vi "plot_displacement.vi"(6 "Position at Peak (decimicrons)":dbl, 7 "Target Pulse Duration (ms)":dbl, 9 "Array":dbl[](array[numeric]), 10 "Array 2":u32[](array[numeric]), 11 "XYGraph in":refnum<vi>) -> (1 "true pulse duration":dbl, 3 "Cluster":cluster{u32[], dbl[]})   [LabVIEW 2014]
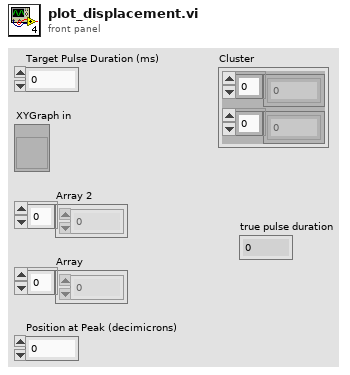
[diagram p1: front panel]
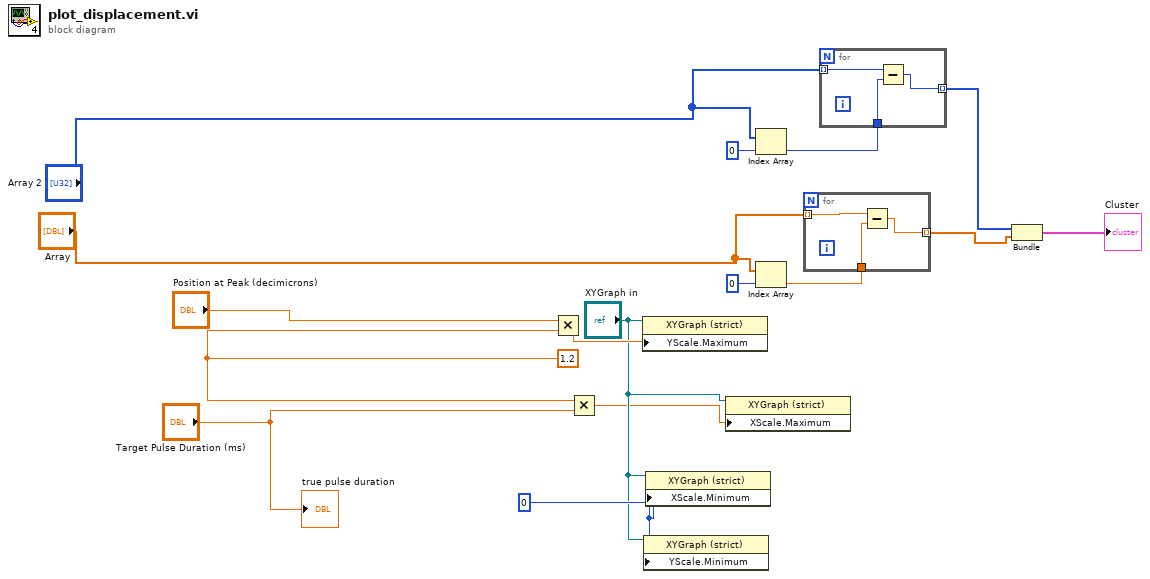
[diagram p0: block diagram]
diagram:
  w7 = 0
  w5 = 1.2
  n1 = Multiply(x="Position at Peak (decimicrons)", y=w5) -> (x*y=w4:dbl)
  n2 = Multiply(x=w5, y="Target Pulse Duration (ms)") -> (x*y=w1:dbl)
  n3 = property on="Property Node" class="XYGraph (strict)"(reference="XYGraph in", "YScale.Maximum"=w4) -> ()  [unwired: 1 in, 2 out]
  n4 = property on="Property Node" class="XYGraph (strict)"(reference="XYGraph in", "YScale.Minimum"=w7) -> ()  [unwired: 1 in, 2 out]
  n5 = property on="Property Node" class="XYGraph (strict)"(reference="XYGraph in", "XScale.Minimum"=w7) -> ()  [unwired: 1 in, 2 out]
  n6 = property on="Property Node" class="XYGraph (strict)"(reference="XYGraph in", "XScale.Maximum"=w1) -> ()  [unwired: 1 in, 2 out]
  n7 = Index Array(array="Array 2", index=0) -> (element=w10:u32)
  n8 = Index Array(array="Array", index=0) -> (element=w13:dbl)
  n9 = for {
    tunnel: [w19] -> w14 mode=indexing
    tunnel: "Array" -> [w18] mode=indexing
    tunnel: w13 -> [w17]
    n10 = Subtract(x=w18, y=w17) -> (x-y=w19:dbl)
  }
  n11 = for {
    tunnel: [w22] -> w15 mode=indexing
    tunnel: "Array 2" -> [w21] mode=indexing
    tunnel: w10 -> [w20]
    n12 = Subtract(x=w21, y=w20) -> (x-y=w22:u32)
  }
  n13 = Bundle(w15, w14) -> (→"Cluster":cluster{u32[], dbl[]})  [unwired: 1 in]
  "true pulse duration" <- "Target Pulse Duration (ms)"
